vi "CVT String Write.vi"(3 "error in (no error)":errorcluster, 4 "Value":string, 5 "Tag Name":string) -> (0 "error out":errorcluster)   [LabVIEW 2020, in "Current Value Table(Rebuild).lvlib"]
uses:
  Current Value Table(Rebuild).lvlib
  DataTypes/String_Write.vi
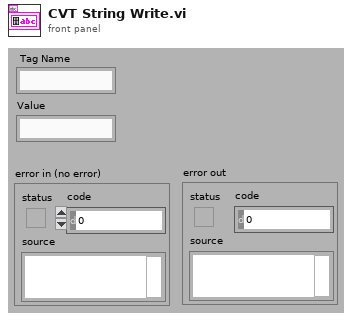
[diagram p1: front panel]
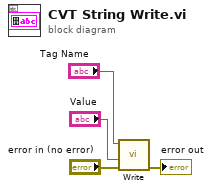
[diagram p0: block diagram]
diagram:
  n1 = call-poly "Write.vi"("error in (no error)"="error in (no error)", "Value"="Value", "Tag Name"="Tag Name") -> ("error out"=→"error out":errorcluster)  [unwired: 8 in]
